vi "Na-DAS_7609.vi"() -> (0 "DAQ Error":errorcluster)   [LabVIEW 2017]
doc: "Use this plug-in with the Nathan 7609 data acquisition system"
uses:
  Globals/Meas_global.vi
  PWA/PWAtasksGLOBAL.vi
  Globals/Extra_Commands_Global.vi
  Globals/Dynamic_call_global.ph.vi
  Globals/Trav_pos_global.vi
panel:
  in  "Minimum timeout (ms)":u32=15000
  in  "Input voltage range (V)":u8(ring)=1 items=["-5... +5 V", "-10... +10 V"]
  out "Config read-back ok":bool
  out "Overruns":u32
  # "Do not close this window between blocks"
  # "PN 25/11/2014, 19/12/2014, 15/02/2015 (channels in any order), 17/08/2015 (stop ack mod), 23/08/2015 (timeout mod for SW vs HW triggering), 03/09/2017 (rising and falling edge options for HW triggering)"
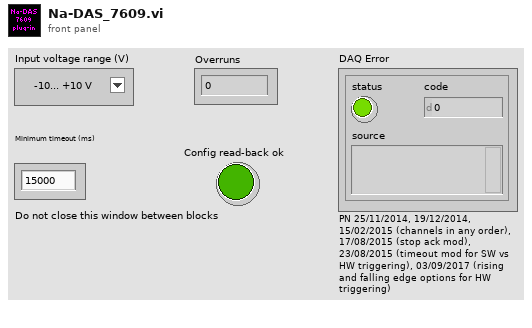
[diagram p1: front panel]
types:
  T1 = typedef "Analysis_info_cluster.ctl" = cluster{"Colour":u32, "Inst type":T2, "Inst name":string, "Symbol":string, "Code name":string, "Extra Info":string, "Inst Array":T3, "Extra Titles":string[], "Extra Values":string[], "U":dbl, "u^2":dbl, "u^3":dbl, "u^4":dbl, "Skew_u":dbl, "Kurt_u":dbl, "Sd Error in Mean":dbl, "% u'/U":dbl, "X":dbl, "Y":dbl, "Z":dbl, "Timescale integral Estimate":dbl, "Sd Error in Variance":dbl, "Calib File":path, "Calib Constants":dbl[], "Output Position":bool, "Full Stats":bool, "Av Sampling Rate":dbl, "Av No of Samples":dbl, "Total Meas Time (s)":dbl, "ADAM Ch Name":string, "Max value":dbl, "Min value":dbl, "Req Sample Rate Hz":dbl, "Sync Delay Time (s)":dbl, "Ch No":i16, "Device ID":string, "Use Latest Calib":bool}
  T2 = typedef "Inst_type.ctl" = enum16{"Propeller anemometer", "Raw voltage", "Pressure Transducer", "Pitot-static tube", "Preston tube", "Hot wire", "Cross wire 1", "Cross wire 2", "Generic Linear", "Generic Polynomial", "Generic BackPoly", "Fast FID", "Thermocouple", "Cold wire", "Pulsed Wire", "LDA Vel", "LDA Tran time", "LDA Arr time", "Microphone"}
  T3 = typedef "Instrument_Array.ctl" = enum16{"PWA", "LDA", "Analogue"}
  T4 = typedef "LDA_Setup.ctl" = cluster{"dimensions":enum16{"1D", "2D"}, "Analogue Freq Multiplier":dbl}
  T5 = typedef "Traverse_cluster.ctl" = cluster{"Start X":sgl, "Start Y":sgl, "Start Z":sgl, "End X":sgl, "End Y":sgl, "End Z":sgl, "No. of pts.":i32, "Spacing":T6, "Filename":path, "Tunnel Speed":dbl, "Averaging time (min)":dbl, "Extra Commands":string, "Carrier_1 Q (l/min)":dbl, "Carrier_2 Q (l/min)":dbl, "Trace Gas Concentration (%)":dbl, "Specific Arguments":string, "Comments":string, "Row No":i32, "Row Type Selector":T7, "Completion time":string, "Row Duration (mins)":dbl, "No. of Valid pts.":i32, "Meas Setup File":string}
  T6 = typedef "Spacing.ctl" = enum16{"Linear", "Log", "Gauss", "Specified", "N/A"}
  T7 = typedef "Multi_run_mode.ctl" = enum16{"Move Traverse Only", "Set Tunnel Speed Only", "Set Source Only", "Set Measurement Conditions", "Single Measurement", "Vertical Profile", "Lateral Profile", "Longitudinal Profile", "Explore Volume", "Multi-Axis Profile", "Auto Calibrate", "Meas Fast FID Bkgnd", "Check Beam Power", "Scanning Valve Measurement", "Run VI Named:", "Set ADAM Ch", "Wait (minutes)", "Send Message", "Synchronize With:", "Fall Back to this Row", "Turn Off Row Repeating", "Blank Row", "Traverse 3D Volume"}
  T8 = typedef "Trigger_Mode.ctl" = enum16{"Free Running", "Start on Trigger", "Trigger Every Block", "Trigger Every Sample"}
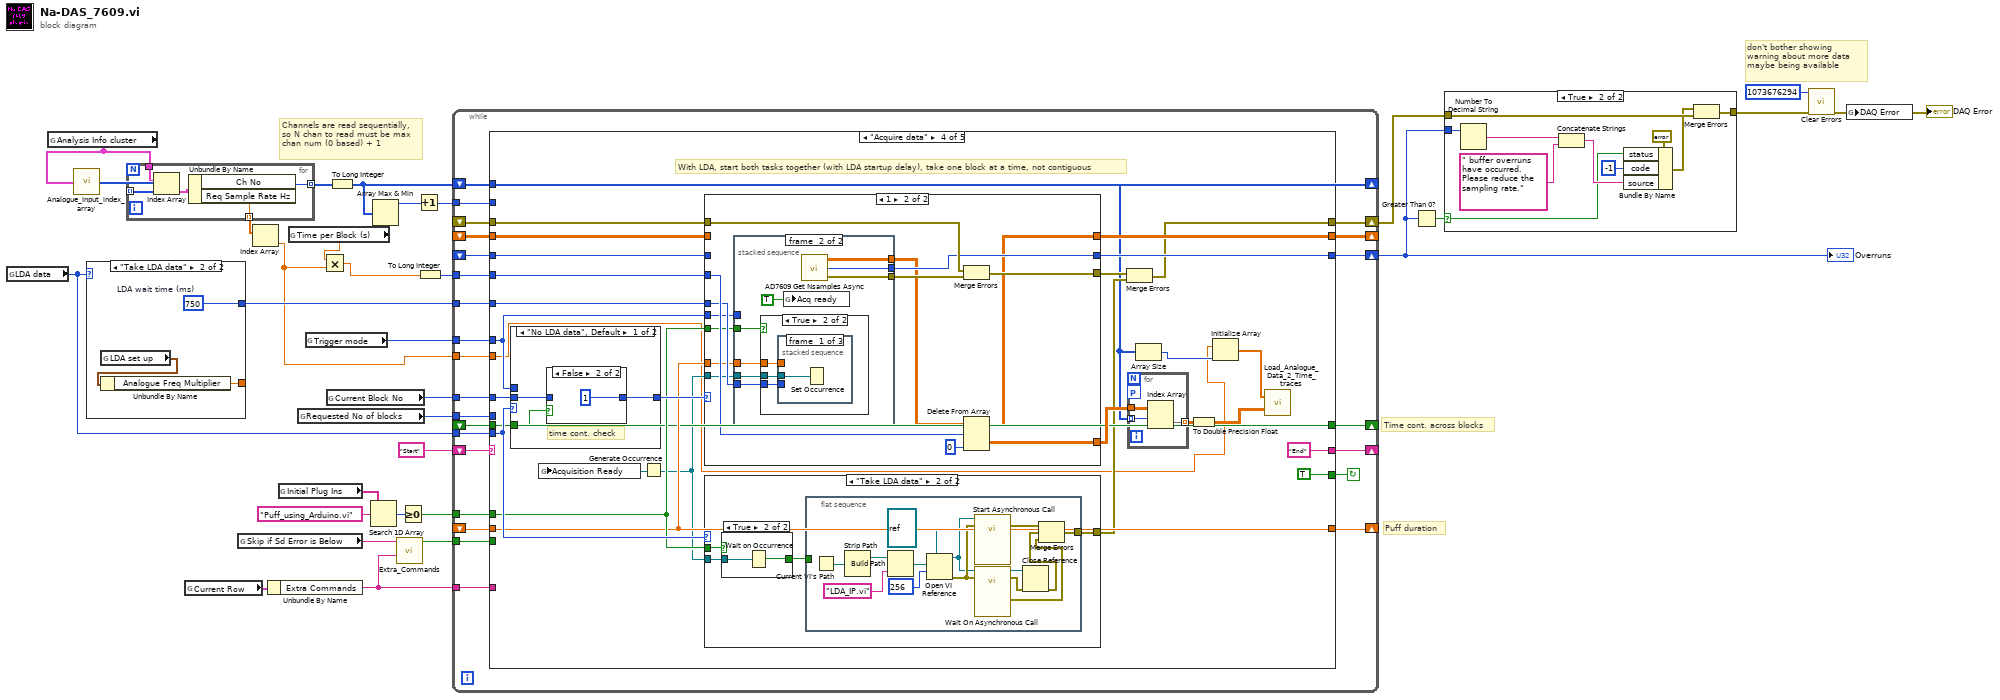
[diagram p0: block diagram]
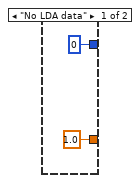
[diagram p3: hidden frame]
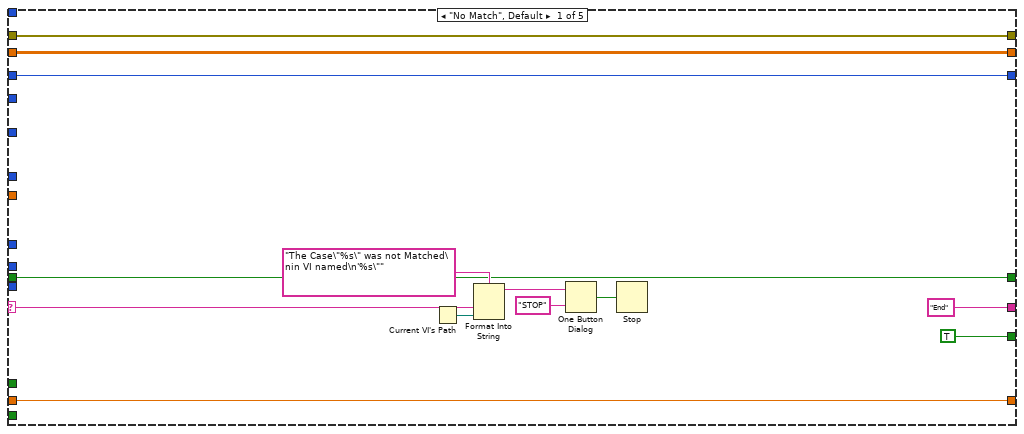
[diagram p4: hidden frame]
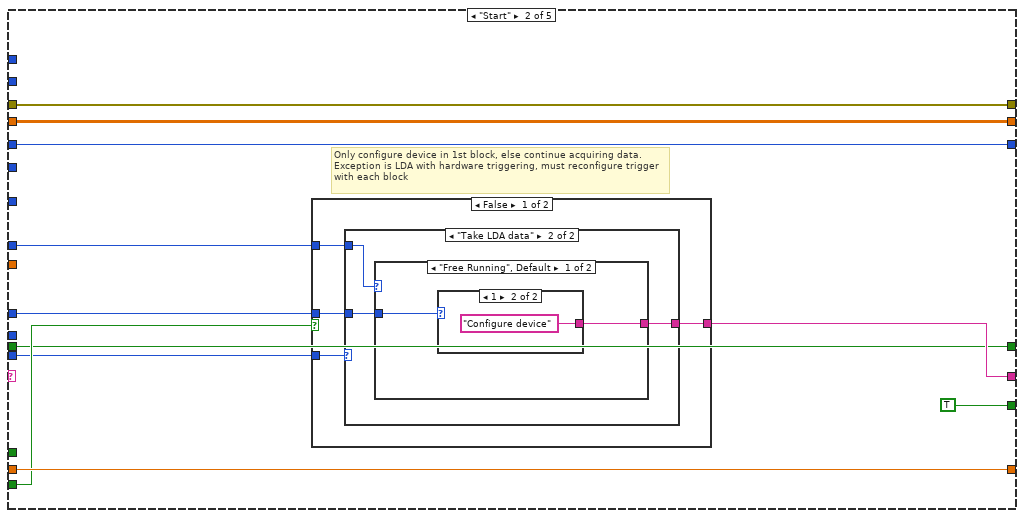
[diagram p5: hidden frame]
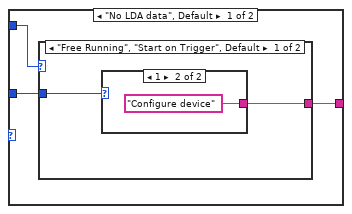
[diagram p6: hidden frame]
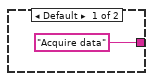
[diagram p7: hidden frame]
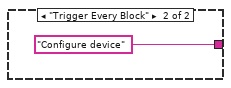
[diagram p8: hidden frame]
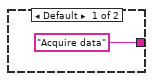
[diagram p9: hidden frame]
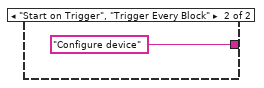
[diagram p10: hidden frame]
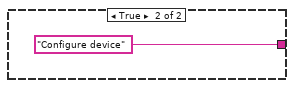
[diagram p11: hidden frame]
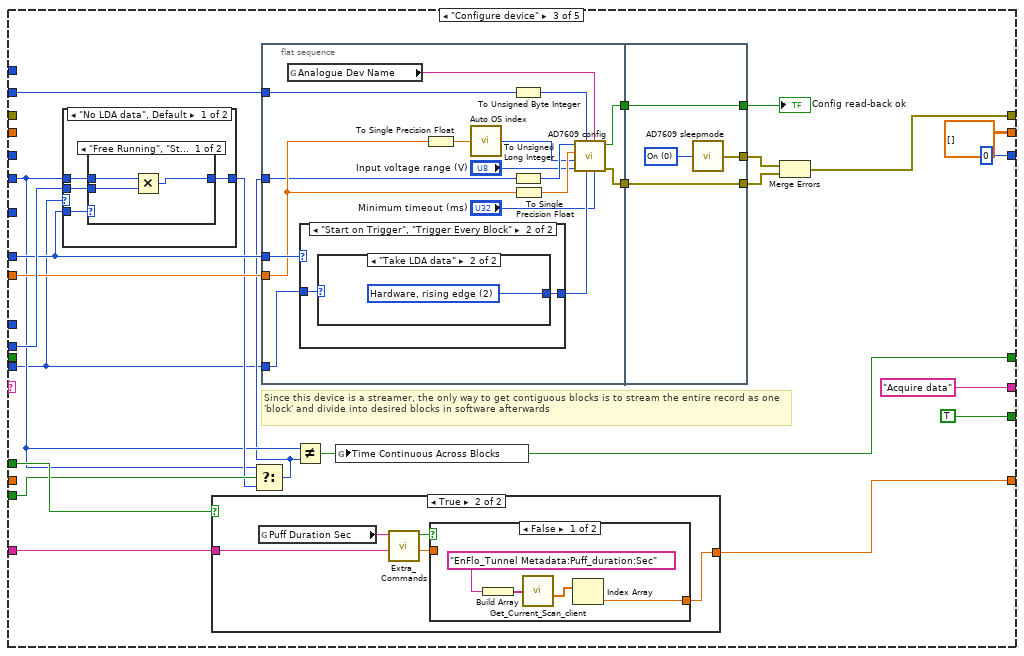
[diagram p12: hidden frame]
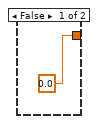
[diagram p13: hidden frame]
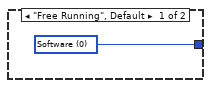
[diagram p17: hidden frame]
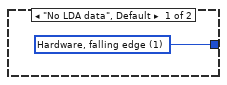
[diagram p18: hidden frame]
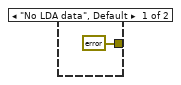
[diagram p19: hidden frame]
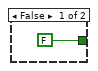
[diagram p20: hidden frame]
diagram:
  # "don't bother showing warning about more data maybe being available"
  # "Time cont. across blocks"
  # "Puff duration"
  # "Channels are read sequentially, so N chan to read must be max chan num (0 based) + 1"
  n1 = global read "Meas_global.vi" "LDA data"() -> (w28:enum16{"No LDA data", "Take LDA data"})
  n2 = global read "Meas_global.vi" "Analysis Info cluster"() -> (w6:T1[])
  n3 = call "Analogue_Input_index_array.vi"("Analysis Info cluster"=w6) -> ("Array"=w5:i32[])
  n4 = case shown="\"Take LDA data\"" w28 {
    tunnel: [1.0 ("Analogue Freq Multiplier") w35] -> _
    tunnel: [u32 0 ("LDA wait time (ms)") w34] -> w23
    frame "No LDA data" {
    }
    frame "Take LDA data" {
      w34 = u32 750  # LDA wait time (ms)
      n5 = global read "Meas_global.vi" "LDA set up"() -> (w36:T4)
      n6 = Unbundle By Name(w36) -> ("Analogue Freq Multiplier"=w35:dbl)
    }
  }
  n7 = for {
    tunnel: [w41] -> w18 mode=indexing
    tunnel: w6 -> [w40]
    tunnel: w5 -> [w39] mode=indexing
    tunnel: [w37] -> w4 mode=indexing
    n8 = Index Array(array=w40, index=w39) -> (element=w38:T1)
    n9 = Unbundle By Name(w38) -> ("Ch No"=w41:i16, "Req Sample Rate Hz"=w37:dbl)
  }
  n10 = global read "Trav_pos_global.vi" "Current Row"() -> (w14:T5)
  n11 = global read "Extra_Commands_Global.vi" "Skip if Sd Error is Below"() -> (w13:string)
  n12 = Index Array(array=w4) -> (element=w2:dbl)  [unwired: 1 in]
  n13 = Unbundle By Name(w14) -> ("Extra Commands"=w12:string)
  n14 = global read "Dynamic_call_global.ph.vi" "Initial Plug Ins"() -> (w25:string[])
  n15 = global read "Meas_global.vi" "Time per Block (s)"() -> (w3:dbl)
  n16 = global read "Meas_global.vi" "Requested No of blocks"() -> (w20:i32)
  n17 = global read "Meas_global.vi" "Trigger mode"() -> (w30:T8)
  n18 = Multiply(x=w3, y=w2) -> (x*y=w1:dbl)
  n19 = global read "Meas_global.vi" "Current Block No"() -> (w29:i32)
  n20 = To Long Integer(number=w18) -> (32bit integer=w17:i32[])
  n21 = Search 1D Array(1D array=w25, element="Puff_using_Arduino.vi") -> (index of element=w27:i32)  [unwired: 1 in]
  n22 = Array Max & Min(array=w17) -> (max value=w16:i32)  [unwired: 3 out]
  n23 = call "Extra_Commands.vi"("String to Search"=w12, "Command"=w13) -> ("Command Found"=w11:bool)  [unwired: 2 in, 3 out]
  n24 = Greater Or Equal To 0?(x=w27) -> (x >= 0?=w24:bool)
  n25 = Increment(x=w16) -> (x+1=w15:i32)
  n26 = To Long Integer(number=w1) -> (32bit integer=w19:i32)
  n27 = while {
    shift-left: "Start" -> [w66]
    shift-right: [w52] -> _
    tunnel: w2 -> [w65]
    tunnel: w19 -> [w64]
    tunnel: w29 -> [w63]
    tunnel: w30 -> [w61]
    tunnel: w28 -> [w60]
    tunnel: w20 -> [w59]
    shift-right: [w57] -> w22
    shift-left: _ -> [w58]
    shift-right: [w56] -> _
    shift-left: _ -> [w55]
    shift-right: [w54] -> w9
    shift-left: _ -> [w53]
    tunnel: w23 -> [w51]
    tunnel: w24 -> [w50]
    shift-right: [w49] -> _
    shift-left: _ -> [w48]
    shift-right: [w47] -> _
    shift-left: w17 -> [w47]
    tunnel: w15 -> [w46]
    tunnel: w12 -> [w45]
    tunnel: w11 -> [w44]
    shift-right: [w43] -> _
    shift-left: _ -> [w42]
    stop <- w62 continue-if-true
    n28 = case shown="\"Acquire data\"" w66 {
      selector: w66 -> [w72 _ _ _ _]
      tunnel: ["End" w87 "Acquire data" ("f") "End" "End" ("f")] -> w52
      tunnel: w65 -> [_ _ w123 w181 _]
      tunnel: w64 -> [_ _ w115 w201 _]
      tunnel: w63 -> [_ w88 _ w197 w284]
      tunnel: [TRUE TRUE TRUE TRUE FALSE] -> w62
      tunnel: w61 -> [_ w80 w122 w192 _]
      tunnel: w60 -> [_ w81 w112 w195 _]
      tunnel: w59 -> [_ _ w132 _ w285]
      tunnel: w58 -> [w71 w89 _ w204 w282]
      tunnel: [w71 w89 w133 w186 w281] -> w57
      tunnel: [w70 w86 sgl[][] [] ("Channel volts") w199 w280] -> w56
      tunnel: w55 -> [w70 w86 _ w200 w280]
      tunnel: [w69 w85 u32 0 ("Overruns") w203 w279] -> w54
      tunnel: w53 -> [w69 w85 _ w202 w279]
      tunnel: w51 -> [_ _ _ w196 _]
      tunnel: w50 -> [_ _ w121 w194 _]
      tunnel: [w68 w84 w120 w193 w278] -> w49
      tunnel: w48 -> [w68 w84 _ w193 w278]
      tunnel: w47 -> [_ _ _ w183 _]
      tunnel: w46 -> [_ _ w119 _ _]
      tunnel: w45 -> [_ _ w118 _ _]
      tunnel: w44 -> [_ w83 w117 _ _]
      tunnel: [w67 w82 w113 w189 w277] -> w43
      tunnel: w42 -> [w67 w82 _ w189 w277]
      frame "No Match", Default {
        n29 = Current VI's Path() -> (path=w75:path)
        n30 = Format Into String(format string="The Case\"%s\" was not Matched\nin VI named\n'%s\"" ("Format String"), w72, w75) -> (resulting string=w78:string)  [unwired: 2 in, 1 out]
        n31 = One Button Dialog(message=w78, button name ("OK")="STOP") -> (true=w76:bool)
        n32 = Stop(stop? (T)=w76) -> ()
      }
      frame "Start" {
        # "Only configure device in 1st block, else continue acquiring data. Exception is LDA with hardware triggering, must reconfigure trigger with each block"
        n33 = case shown="False" w83 {
          tunnel: w88 -> [w94 _]
          tunnel: [w93 "Configure device" ("f")] -> w87
          tunnel: w81 -> [w92 _]
          tunnel: w80 -> [w91 _]
          frame False {
            n34 = case shown="\"Take LDA data\"" w92 {
              tunnel: w94 -> [w97 w103]
              tunnel: [w96 w104] -> w93
              tunnel: w91 -> [w95 w105]
              frame "No LDA data", Default {
                n35 = case shown="\"Free Running\", \"Start on Trigger\", Default" w95 {
                  tunnel: w97 -> [w99 _]
                  tunnel: [w98 "Configure device" ("f")] -> w96
                  frame "Free Running", "Start on Trigger", Default {
                    n36 = case shown="1" w99 {
                      tunnel: ["Acquire data" ("f") "Configure device" ("f")] -> w98
                      frame Default {
                      }
                      frame 1 {
                      }
                    }
                  }
                  frame "Trigger Every Block" {
                  }
                }
              }
              frame "Take LDA data" {
                n37 = case shown="\"Free Running\", Default" w105 {
                  tunnel: [w107 "Configure device" ("f")] -> w104
                  tunnel: w103 -> [w106 _]
                  frame "Free Running", Default {
                    n38 = case shown="1" w106 {
                      tunnel: ["Acquire data" ("f") "Configure device" ("f")] -> w107
                      frame Default {
                      }
                      frame 1 {
                      }
                    }
                  }
                  frame "Start on Trigger", "Trigger Every Block" {
                  }
                }
              }
            }
          }
          frame True {
          }
        }
      }
      frame "Configure device" {
        # "Since this device is a streamer, the only way to get contiguous blocks is to stream the entire record as one 'block' and divide into desired blocks in software afterwards"
        n39 = case shown="\"No LDA data\", Default" w112 {
          tunnel: [w147 w154] -> w116
          tunnel: w115 -> [w149 w154]
          tunnel: w132 -> [w148 _]
          tunnel: w122 -> [w146 _]
          frame "No LDA data", Default {
            n40 = case shown="\"Free Running\", \"Start on Trigger\", Default" w146 {
              tunnel: w149 -> [w152 w153]
              tunnel: w148 -> [w151 _]
              tunnel: [w150 w153] -> w147
              frame "Free Running", "Start on Trigger", Default {
                n41 = Multiply(x=w152, y=w151) -> (x*y=w150:i32)
              }
              frame "Trigger Every Block" {
              }
            }
          }
          frame "Take LDA data" {
          }
        }
        n42 = case shown="True" w121 {
          tunnel: [0.0 w140] -> w120
          tunnel: w118 -> [_ w136]
          frame False {
          }
          frame True {
            n43 = global read "Extra_Commands_Global.vi" "Puff Duration Sec"() -> (w139:string)
            n44 = call "Extra_Commands.vi"("String to Search"=w136, "Command"=w139) -> ("Numeric Value"=w137:dbl, "Command Found"=w138:bool)  [unwired: 2 in, 2 out]
            n45 = case shown="False" w138 {
              tunnel: [w141 w145] -> w140
              tunnel: w137 -> [_ w145]
              frame False {
                n46 = Build Array("EnFlo_Tunnel Metadata:Puff_duration:Sec") -> (w143:string[])
                n47 = call "Get_Current_Scan_client.vi"("ADAM Ch Names"=w143) -> ("Numerical Values"=w144:dbl[])  [unwired: 1 in, 2 out]
                n48 = Index Array(array=w144) -> (element=w141:dbl)  [unwired: 1 in]
              }
              frame True {
              }
            }
          }
        }
        n49 = Select(t=w115, s=w117, f=w116) -> (s? t:f=w114:i32)
        n50 = flat-sequence {
          tunnel: w114 -> [w155]
          tunnel: w123 -> [w161]
          tunnel: w122 -> [w170]
          tunnel: [w164] -> w131
          tunnel: [w163] -> w130
          tunnel: w119 -> [w158]
          tunnel: w112 -> [w156]
          tunnel: [w178] -> w127
          tunnel: w131 -> [w178]
          tunnel: [w177] -> w129
          tunnel: w130 -> [w177]
          tunnel: [w176] -> w128
          frame #0 {
            n51 = global read "PWAtasksGLOBAL.vi" "Analogue Dev Name"() -> (w169:string)
            n52 = case shown="\"Start on Trigger\", \"Trigger Every Block\"" w170 {
              tunnel: [w171 w173] -> w166
              tunnel: w156 -> [_ w172]
              frame "Free Running", Default {
                w171 = u8 0 items=["Software", "Hardware, falling edge", "Hardware, rising edge"] ("Triggering mode")
              }
              frame "Start on Trigger", "Trigger Every Block" {
                n53 = case shown="\"Take LDA data\"" w172 {
                  tunnel: [w174 w175] -> w173
                  frame "No LDA data", Default {
                    w174 = u8 1 items=["Software", "Hardware, falling edge", "Hardware, rising edge"] ("Triggering mode")
                  }
                  frame "Take LDA data" {
                    w175 = u8 2 items=["Software", "Hardware, falling edge", "Hardware, rising edge"] ("Triggering mode")
                  }
                }
              }
            }
            n54 = To Single Precision Float(number=w161) -> (single precision float=w159:sgl)
            n55 = call "Auto OS index.vi"("Sampling rate"=w159) -> ("OS index"=w160:u8)
            n56 = To Unsigned Byte Integer(number=w158) -> (unsigned 8bit integer=w165:u8)
            n57 = To Unsigned Long Integer(number=w155) -> (unsigned 32bit integer=w168:u32)
            n58 = To Single Precision Float(number=w161) -> (single precision float=w167:sgl)
            n59 = call "AD7609 config.vi"("Timeout for software trig. mode (ms)"="Minimum timeout (ms)", "Device serial port"=w169, "Triggering mode"=w166, "N channels to read"=w165, "Input voltage range (V)"="Input voltage range (V)", "Oversampling ratio"=w160, "Sampling rate (Hz)"=w167, "Number of samples"=w168) -> ("Config error out"=w163:errorcluster, "Config read-back ok"=w164:bool)  [unwired: 2 in]
          }
          frame #1 {
            w179 = u8 0 items=["On", "Standby", "Shutdown"] ("Sleep state")
            n60 = call "AD7609 sleepmode.vi"("Sleep state"=w179) -> ("Sleep error out"=w176:errorcluster)
          }
        }
        n61 = Not Equal?(x=w115, y=w114) -> (x != y?=w113:bool)
        n62 = global write "Meas_global.vi" "Time Continuous Across Blocks"(w113) -> ()
        n63 = Merge Errors(w128, w129) -> (w133:errorcluster)
        "Config read-back ok" <- w127
      }
      frame "Acquire data" {
        # "With LDA, start both tasks together (with LDA startup delay), take one block at a time, not contiguous"
        n64 = case shown="\"No LDA data\", Default" w195 {
          tunnel: w197 -> [w233 _]
          tunnel: w192 -> [_ _]
          tunnel: [w234 1 ("Current Block No")] -> w198
          tunnel: w189 -> [w232 _]
          frame "No LDA data", Default {
            # "time cont. check"
            n65 = case shown="False" w232 {
              tunnel: [w235 1 ("Current Block No")] -> w234
              tunnel: w233 -> [w235 _]
              frame True {
              }
              frame False {
              }
            }
          }
          frame "Take LDA data" {
          }
        }
        n66 = Generate Occurrence() -> (w185:refnum<k4>)
        n67 = global write "Meas_global.vi" "Acquisition Ready"(w185) -> ()
        n68 = case shown="1" w198 {
          tunnel: w204 -> [w239 w257]
          tunnel: [w239 w256] -> w188
          tunnel: [w240 w255] -> w203
          tunnel: [w242 w252] -> w199
          tunnel: w201 -> [w241 w253]
          tunnel: w200 -> [w243 _]
          tunnel: w202 -> [w240 _]
          tunnel: [w238 w250] -> w191
          tunnel: w196 -> [_ w249]
          tunnel: w185 -> [_ w248]
          tunnel: w194 -> [_ w247]
          tunnel: w193 -> [_ w246]
          tunnel: w192 -> [_ w245]
          frame Default {
            # "First block gets ALL samples (N_blocks * samples per block). Output one block of samples and keep remainder for next block cycle."
            n69 = Delete From Array(array=w243, length=w241, index (col)=0 ("disabled index (col)")) -> (deleted portion=w238:sgl[][], array with subset deleted=w242:sgl[][])  [unwired: 1 in]
          }
          frame 1 {
            n70 = stacked-sequence {
              tunnel: [_ w268] -> w255
              tunnel: [_ w267] -> w254
              tunnel: [_ w266] -> w258
              tunnel: w248 -> [_ w265]
              tunnel: w249 -> [w260 w264]
              tunnel: w247 -> [_ w263]
              tunnel: w246 -> [_ w262]
              tunnel: w245 -> [w259 _]
              frame #0 {
                n71 = case shown="\"Free Running\"" w259 {
                  tunnel: w260 -> [w261 _]
                  frame "Free Running" {
                    n72 = Wait (ms)(milliseconds to wait=w261) -> ()  [unwired: 1 out]
                  }
                  frame Default {
                  }
                }
              }
              frame #1 {
                n73 = case shown="True" w263 {
                  tunnel: w265 -> [w270 w273]
                  tunnel: w262 -> [_ w272]
                  tunnel: w264 -> [_ w271]
                  frame False {
                    n74 = Set Occurrence(w270) -> ()
                  }
                  frame True {
                    n75 = stacked-sequence {
                      tunnel: w273 -> [w274 _ _]
                      tunnel: w272 -> [_ _ w276]
                      tunnel: w271 -> [_ w275 _]
                      frame #0 {
                        n76 = Set Occurrence(w274) -> ()
                      }
                      frame #1 {
                        n77 = Wait (ms)(milliseconds to wait=w275) -> ()  [unwired: 1 out]
                      }
                      frame #2 {
                        n78 = call "Puff_using_Arduino_oneshot.vi"("Puff_duration:Sec"=w276) -> ()  [unwired: 7 in]
                      }
                    }
                  }
                }
                n79 = global write "Meas_global.vi" "Acq ready"(TRUE ("Acq ready")) -> ()
                n80 = call "AD7609 Get Nsamples Async.vi"() -> ("Channel volts"=w267:sgl[][], "Overruns"=w268:u32, "Async error"=w266:errorcluster)  [unwired: 1 in]
              }
            }
            n81 = Merge Errors(w257, w258) -> (w256:errorcluster)
            n82 = Delete From Array(array=w254, length=w253, index (col)=0 ("disabled index (col)")) -> (deleted portion=w250:sgl[][], array with subset deleted=w252:sgl[][])  [unwired: 1 in]
          }
        }
        n83 = case shown="\"Take LDA data\"" w195 {
          tunnel: w194 -> [_ w214]
          tunnel: w185 -> [_ w212]
          tunnel: [errorcluster {"status"=FALSE, "code"=0, "source"=""} ("error IO") w211] -> w187
          frame "No LDA data", Default {
          }
          frame "Take LDA data" {
            n84 = case shown="True" w214 {
              tunnel: w212 -> [_ w217]
              tunnel: [FALSE ("timed out") w216] -> w213
              frame False {
              }
              frame True {
                n85 = Wait on Occurrence(2:w217) -> (0:w216:bool)  [unwired: 2 in]
              }
            }
            n86 = flat-sequence {
              tunnel: w213 -> [_]
              tunnel: [w219] -> w211
              frame #0 {
                n87 = Current VI's Path() -> (path=w229:path)
                n88 = Strip Path(path=w229) -> (stripped path=w228:path)  [unwired: 1 out]
                n89 = Build Path(base path=w228, name or relative path="LDA_IP.vi") -> (appended path=w230:path)
                n90 = Open VI Reference(type specifier VI Refnum (for type only)=refnum<vi> refnum, vi path=w230, options=256) -> (vi reference=w224:refnum<vi>, error out=w225:errorcluster)  [unwired: 3 in]
                n91 = call-by-ref "Start Asynchronous Call"(reference=w224, error in=w225) -> (error out=w221:errorcluster)  [unwired: 1 in, 2 out]
                n92 = call-by-ref "Wait On Asynchronous Call"(reference=w224, error in=w225) -> (reference out=w223:refnum<vi>, error out=w222:errorcluster, 0:"error out"=w218:errorcluster)  [unwired: 1 in]
                n93 = Close Reference(reference=w223, error in (no error)=w222) -> (error out=w220:errorcluster)
                n94 = Merge Errors(w221, w220, w218) -> (w219:errorcluster)
              }
            }
          }
        }
        n95 = Merge Errors(w188, w187) -> (w186:errorcluster)
        n96 = for {
          tunnel: w183 -> [w208] mode=indexing
          tunnel: [w207] -> w190 mode=indexing
          workers-P: _ -> [_]
          tunnel: w191 -> [w209]
          n97 = Index Array(array=w209, index (row)=w208) -> (element=w207:sgl[])  [unwired: 1 in]
        }
        n98 = Array Size(array=w183) -> (size(s)=w182:i32)
        n99 = To Double Precision Float(number=w190) -> (double precision float=w184:dbl[][])
        n100 = Initialize Array(w181, w182) -> (w180:dbl[])
        n101 = call "Load_Analogue_Data_2_Time_traces.vi"("Voltage Array"=w184, "Sampling Rate (Hz)"=w180) -> ()  [unwired: 1 in]
      }
      frame "End" {
        n102 = Equal?(x=w284, y=w285) -> (x = y?=w283:bool)
        n103 = case shown="True" w283 {
          tunnel: w282 -> [w289 w291]
          tunnel: [w289 w290] -> w281
          frame False {
          }
          frame True {
            w293 = u8 1 items=["On", "Standby", "Shutdown"] ("Sleep state")
            n104 = call "AD7609 sleepmode.vi"("Sleep state"=w293) -> ("Sleep error out"=w292:errorcluster)
            n105 = Merge Errors(w291, w292) -> (w290:errorcluster)
          }
        }
        n106 = global write "Meas_global.vi" "Acq ready"(FALSE ("Acq ready")) -> ()
      }
    }
  }
  "Overruns" <- w9
  n107 = Greater Than 0?(x=w9) -> (x > 0?=w10:bool)
  n108 = case shown="True" w10 {
    selector: w10 -> [_ w296]
    tunnel: w22 -> [w294 w303]
    tunnel: [w294 w304] -> w21
    tunnel: w9 -> [_ w302]
    frame False {
    }
    frame True {
      n109 = Number To Decimal String(number=w302) -> (decimal integer string=w300:string)  [unwired: 1 in]
      n110 = Concatenate Strings(w300, " buffer overruns have occurred. Please reduce the sampling rate.") -> (w298:string)
      n111 = Bundle By Name(cluster=errorcluster {"status"=FALSE, "code"=0, "source"=""} ("error IO"), "status"=w296, "code"=-1, "source"=w298) -> (w295:errorcluster)
      n112 = Merge Errors(w295, w303) -> (w304:errorcluster)
    }
  }
  n113 = call <vilib>:"Clear Errors.vi"("error in (no error)"=w21, "specific error code to clear (0: all)"=1073676294) -> ("error out"=w8:errorcluster)  [unwired: 4 in, 1 out]
  "DAQ Error" <- w8
  n114 = global write "Meas_global.vi" "DAQ Error"(w8) -> ()
